vi "EMG.vi"(8 "error in":errorcluster, 11 "queue in":T1) -> (0 "error out":errorcluster, 3 "queue out":T1)   [LabVIEW 2011]
panel:
  in  "转盘运动":T2
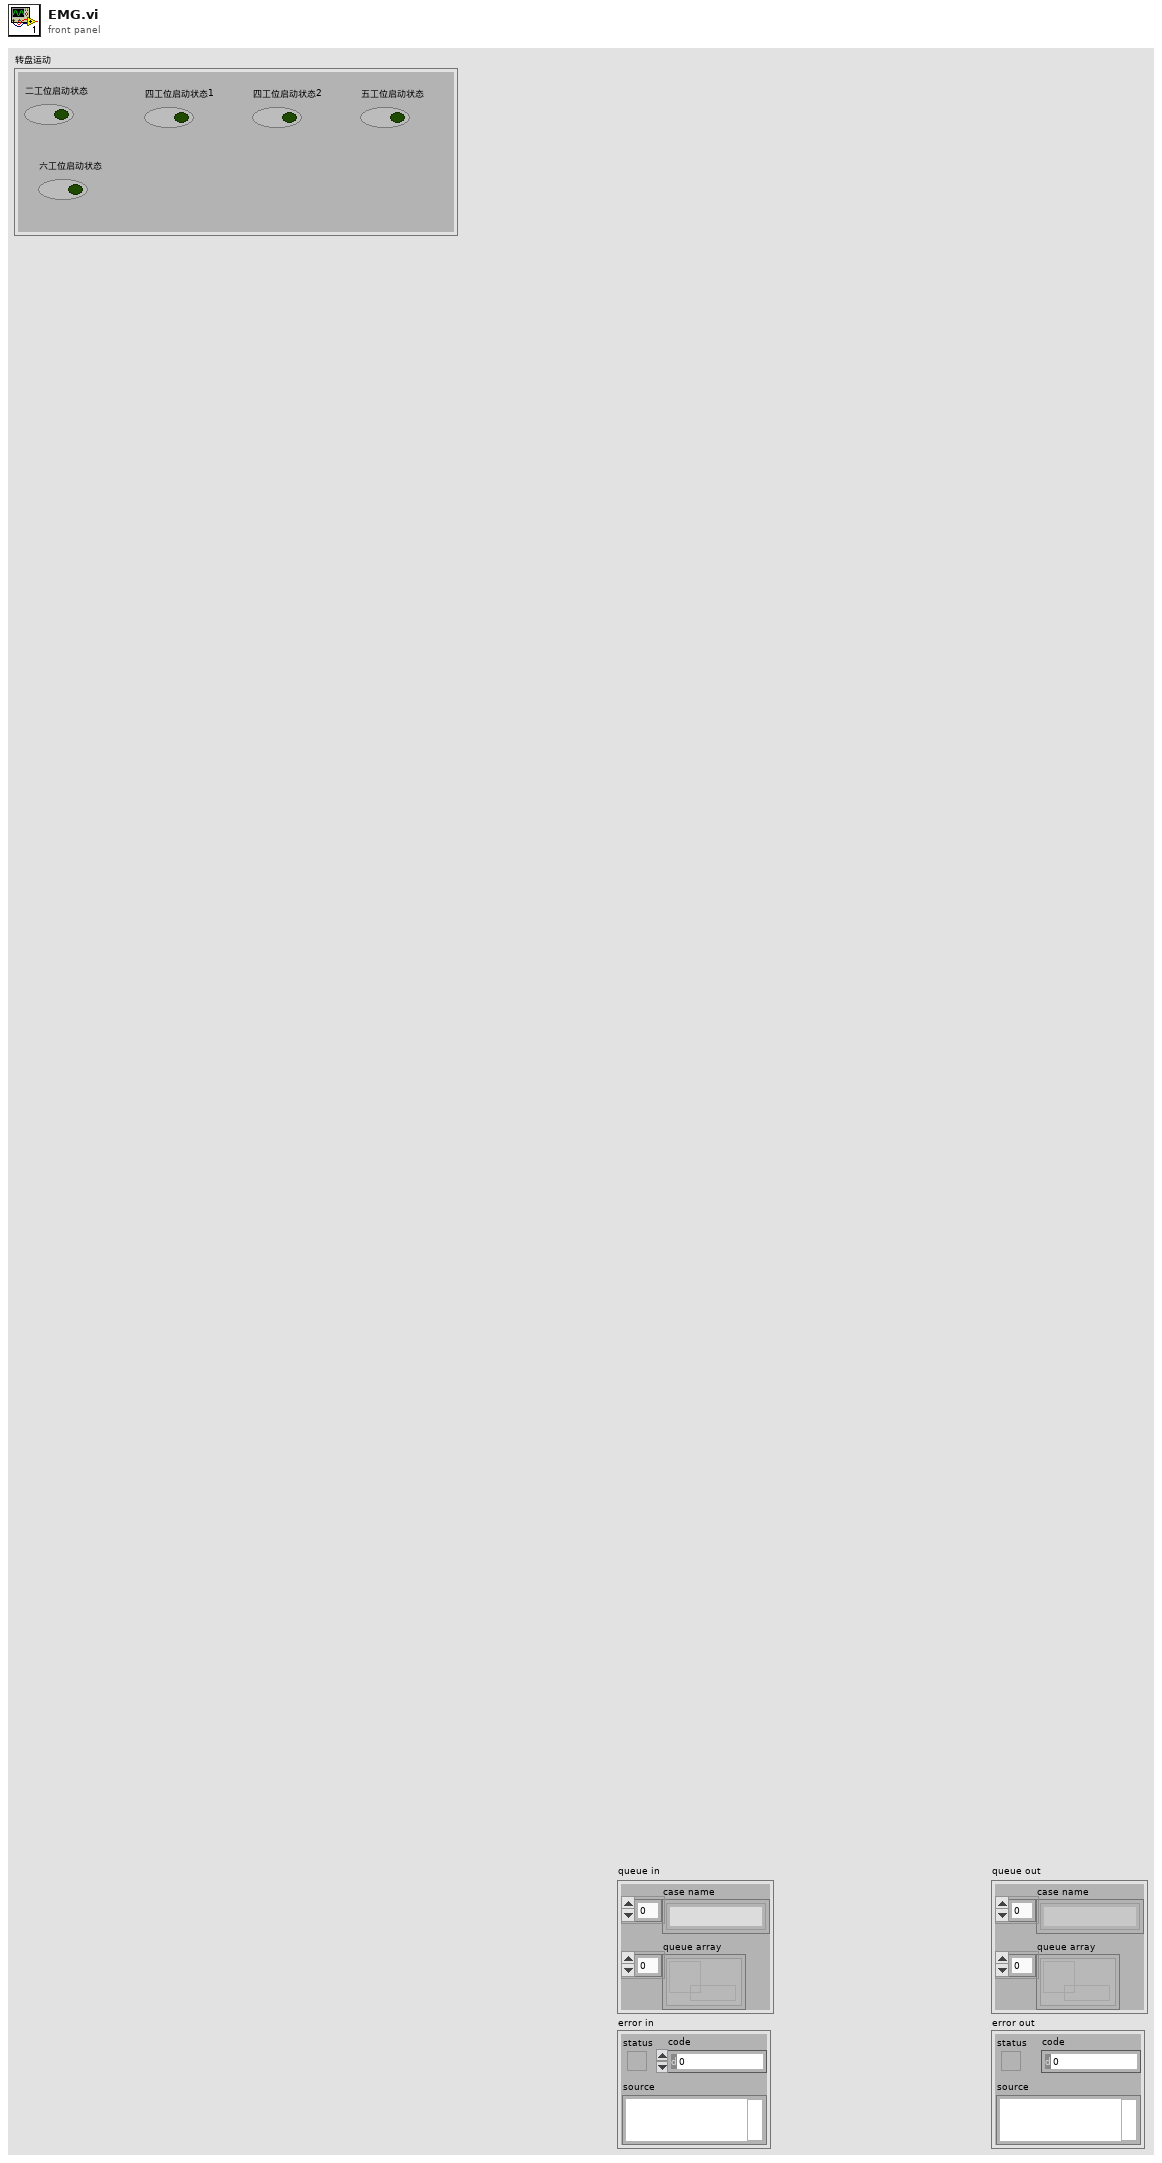
[diagram p1: front panel]
types:
  T1 = cluster{"case name":string[], "queue array":refnum<queue>[]}
  T2 = cluster{"二工位启动状态":bool, "四工位启动状态1":bool, "四工位启动状态2":bool, "五工位启动状态":bool, "六工位启动状态":bool}
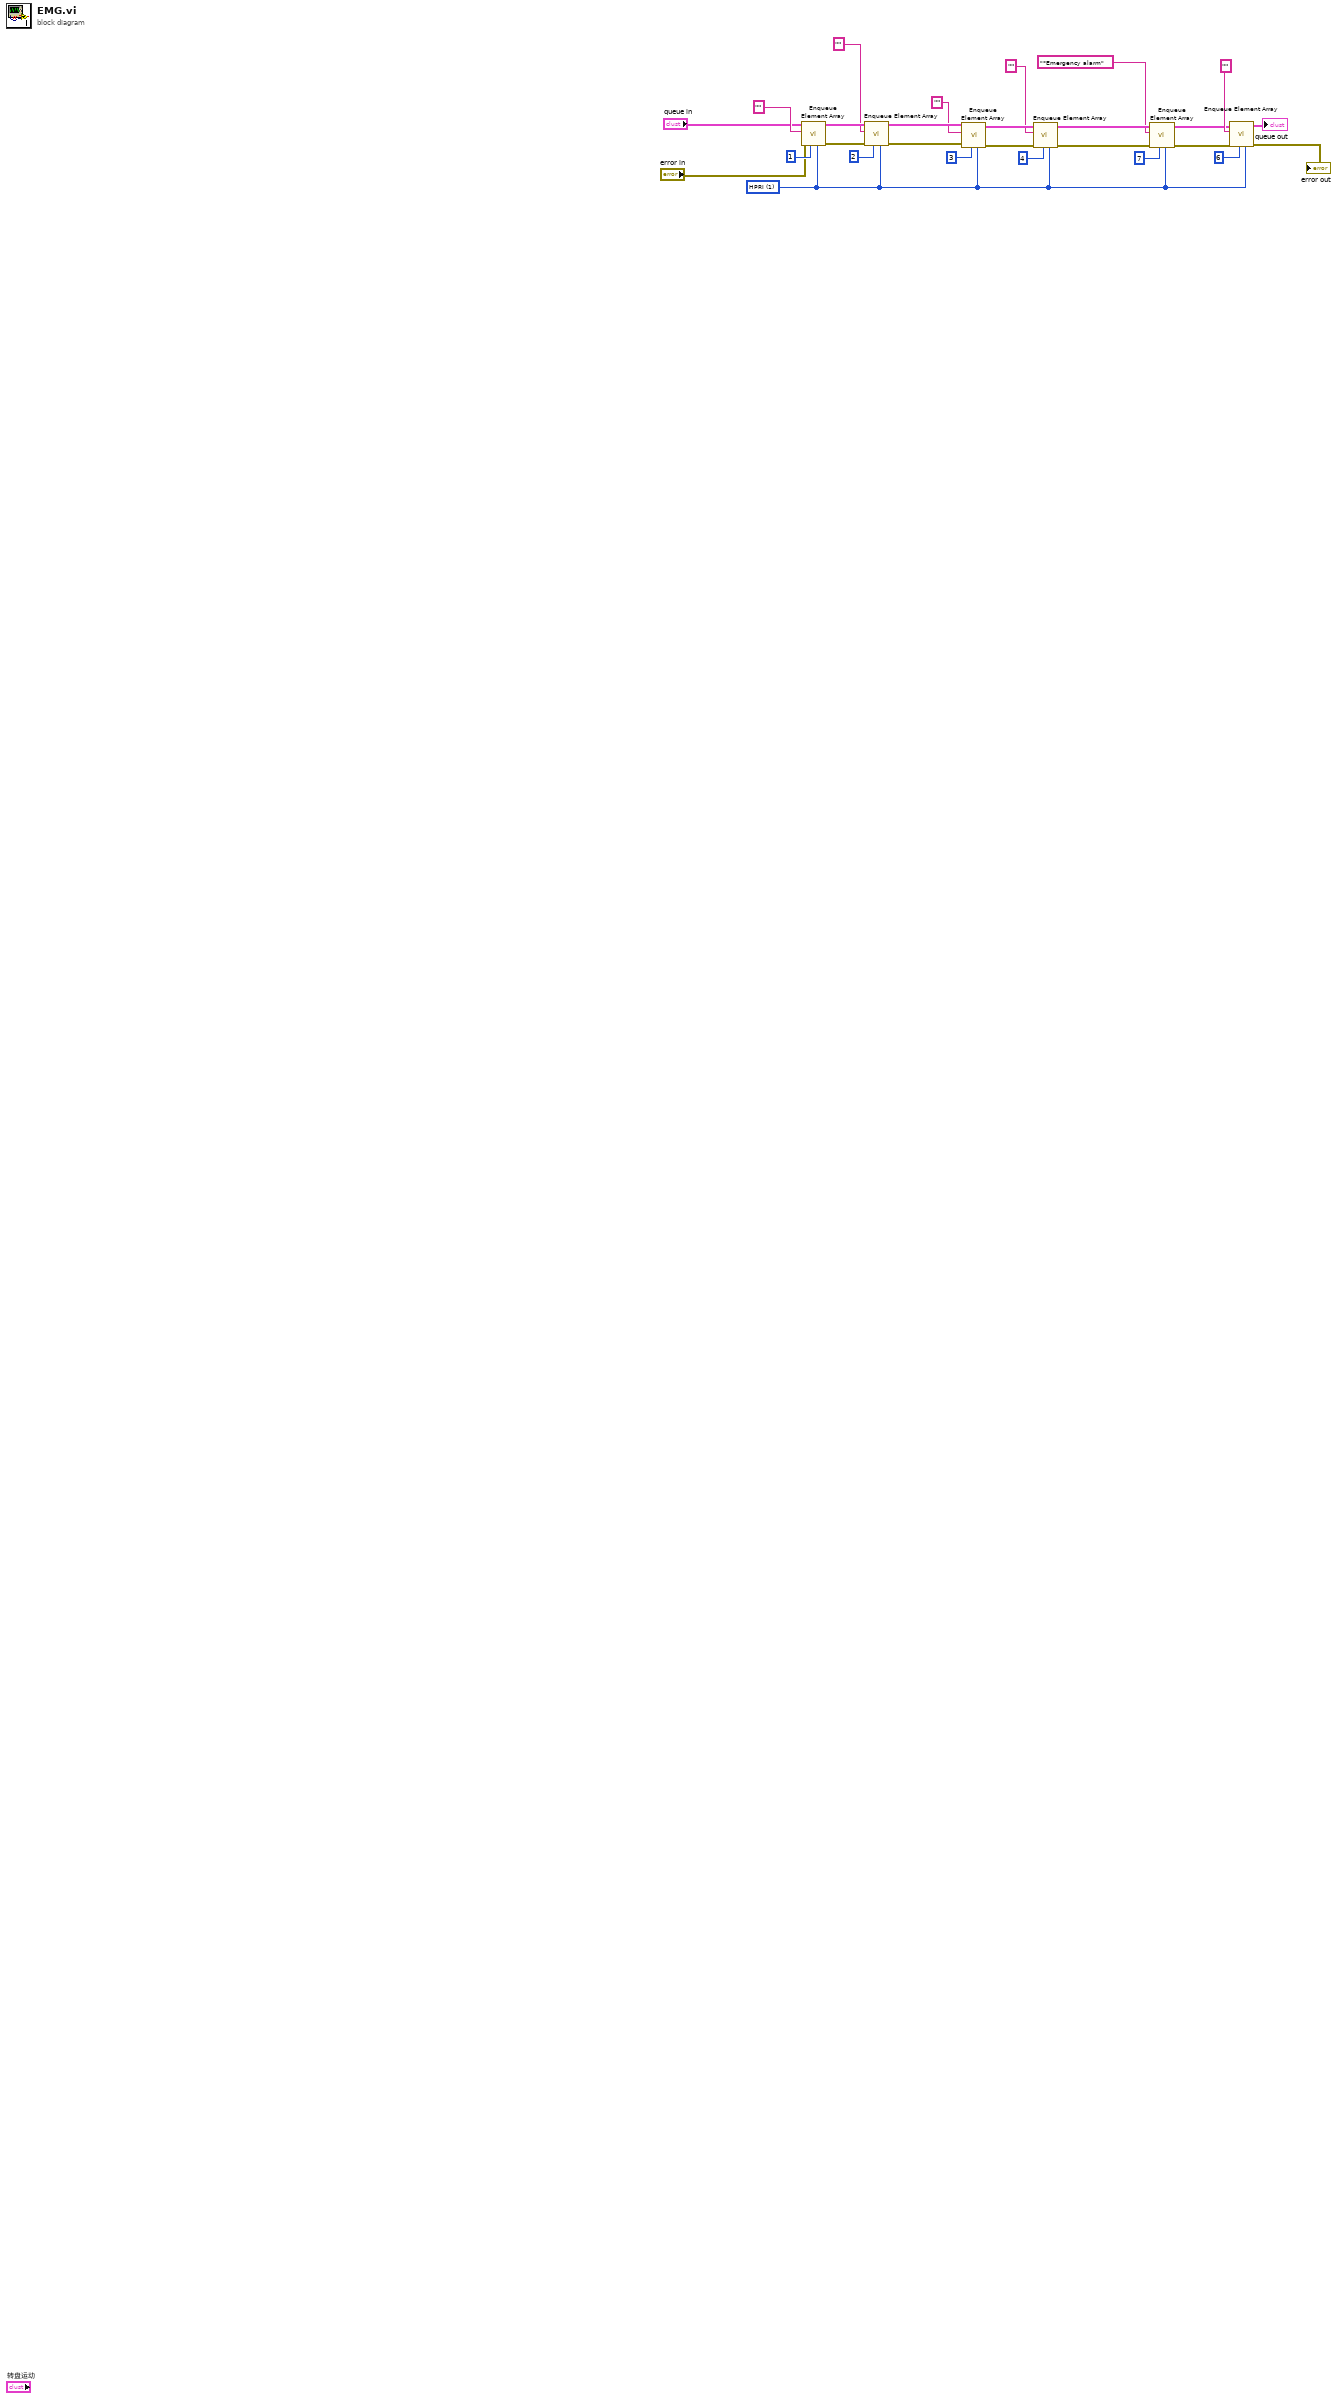
[diagram p0: block diagram]
diagram:
  w1 = u16 1 items=["HPRI"=1, "LPRI"=0] ("priority")
  n1 = call "Enqueue Element Array.vi"("priority"=w1, "queue index"=1, "error in"="error in", "master data"="", "queue in"="queue in") -> ("error out"=w24:errorcluster, "queue out"=w25:T1)  [unwired: 5 in]
  n2 = call "Enqueue Element Array.vi"("priority"=w1, "queue index"=2, "error in"=w24, "master data"="", "queue in"=w25) -> ("error out"=w22:errorcluster, "queue out"=w21:T1)  [unwired: 5 in]
  n3 = call "Enqueue Element Array.vi"("priority"=w1, "queue index"=3, "error in"=w22, "master data"="", "queue in"=w21) -> ("error out"=w20:errorcluster, "queue out"=w19:T1)  [unwired: 5 in]
  n4 = call "Enqueue Element Array.vi"("priority"=w1, "queue index"=4, "error in"=w20, "master data"="", "queue in"=w19) -> ("error out"=w5:errorcluster, "queue out"=w6:T1)  [unwired: 5 in]
  n5 = call "Enqueue Element Array.vi"("priority"=w1, "queue index"=7, "error in"=w5, "master data"="*Emergency alarm", "queue in"=w6) -> ("error out"=w2:errorcluster, "queue out"=w3:T1)  [unwired: 5 in]
  n6 = call "Enqueue Element Array.vi"("priority"=w1, "queue index"=6, "error in"=w2, "master data"="", "queue in"=w3) -> ("error out"=→"error out":errorcluster, "queue out"=→"queue out":T1)  [unwired: 5 in]
